vi "8q_kill CLR.vi"(10 "nextX in":i32[](array[numeric]), 11 "queen in":i32[](array[numeric])) -> (2 "nextX":i32[](array[numeric]), 3 "queen":i32[](array[numeric]))   [LabVIEW 2012]
panel:
  out "array w/ subset deleted":i32[](array[numeric])
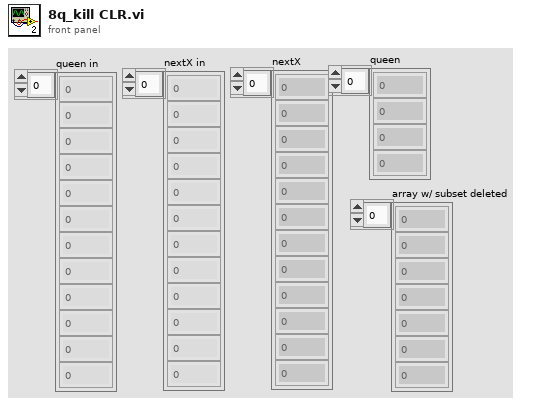
[diagram p1: front panel]
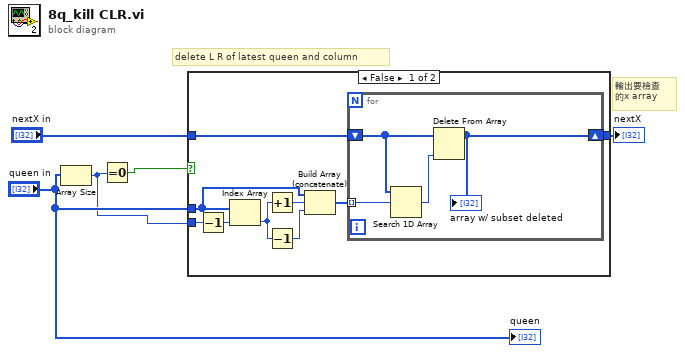
[diagram p0: block diagram]
diagram:
  # "delete L R of latest queen and column"
  # "輸出要檢查\n的x array"
  n1 = Array Size(array="queen in") -> (size(s)=w2:i32)
  n2 = Equal To 0?(x=w2) -> (x = 0?=w1:bool)
  n3 = case shown="False" w1 {
    tunnel: [w10 w19] -> w5
    tunnel: "queen in" -> [w8 _]
    tunnel: "nextX in" -> [w7 w19]
    tunnel: w2 -> [w6 _]
    frame False {
      n4 = Decrement(x=w6) -> (x-1=w9:i32)
      n5 = Index Array(array=w8, index=w9) -> (element=w12:i32)
      n6 = Increment(x=w12) -> (x+1=w14:i32)
      n7 = Decrement(x=w12) -> (x-1=w13:i32)
      n8 = Build Array (concatenate)(w8, w14, w13) -> (w11:i32[])
      n9 = for {
        tunnel: w11 -> [w18] mode=indexing
        shift-right: [w15] -> w10
        shift-left: w7 -> [w16]
        n10 = Search 1D Array(1D array=w16, element=w18) -> (index of element=w17:i32)  [unwired: 1 in]
        n11 = Delete From Array(array=w16, index=w17) -> (array with subset deleted=w15:i32[])  [unwired: 1 in, 1 out]
        "array w/ subset deleted" <- w15
      }
    }
    frame True {
    }
  }
  "nextX" <- w5
  "queen" <- "queen in"
